vi "svx_Colormap Order lines.vi"(4 "pen":T1={"Width"=1, "Style"=enum."Solid"}, 5 "Order":dbl, 6 "color(black)":u32(colorbox), 7 "plot type":T2(ring), 8 "speed profile":cluster{"time [s]":dbl[], "speed [rpm]":dbl[]} {"speed [rpm]" format="%.2f"; "time [s]" format="%.2f"}, 9 "Range":T4, 10 "Plot area":T3, 11 "picture in":picture) -> (0 "End":cluster{"x":i16, "y":i16}, 2 "Begin":cluster{"x":i16, "y":i16}, 3 "picture out":picture)   [LabVIEW 2017, in "SVX Colormap.xctl"]
uses:
  <vilib>/addons/_XControls/Colormap/SVX Colormap.xctl
  <vilib>/Utility/miscctls.llb/LVBoundsTypeDef.ctl
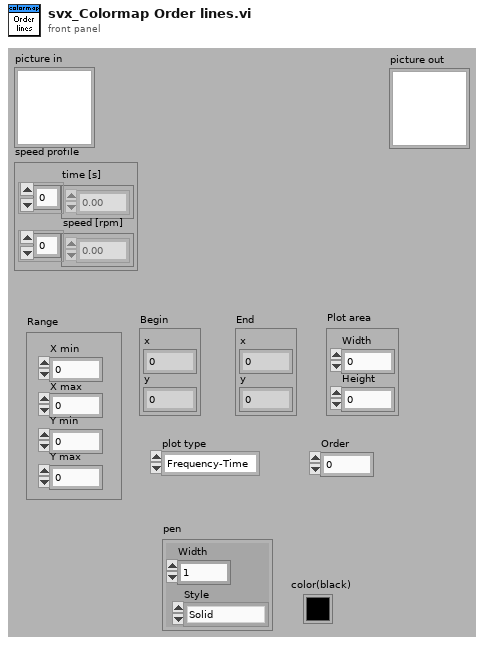
[diagram p1: front panel]
types:
  T1 = cluster{"Width":u16, "Style":enum32{"Solid", "Dash", "Dot", "DashDot", "DashDotDot"}}
  T2 = enum16{"Frequency-Time", "Time-Frequency", "Order-Time", "Time-Order", "Frequency-RPM", "RPM-Frequency", "Order-RPM", "RPM-Order"}
  T3 = typedef "LVBoundsTypeDef.ctl" = cluster{"Width":u32, "Height":u32}
  T4 = cluster{"X min":dbl, "X max":dbl, "Y min":dbl, "Y max":dbl}
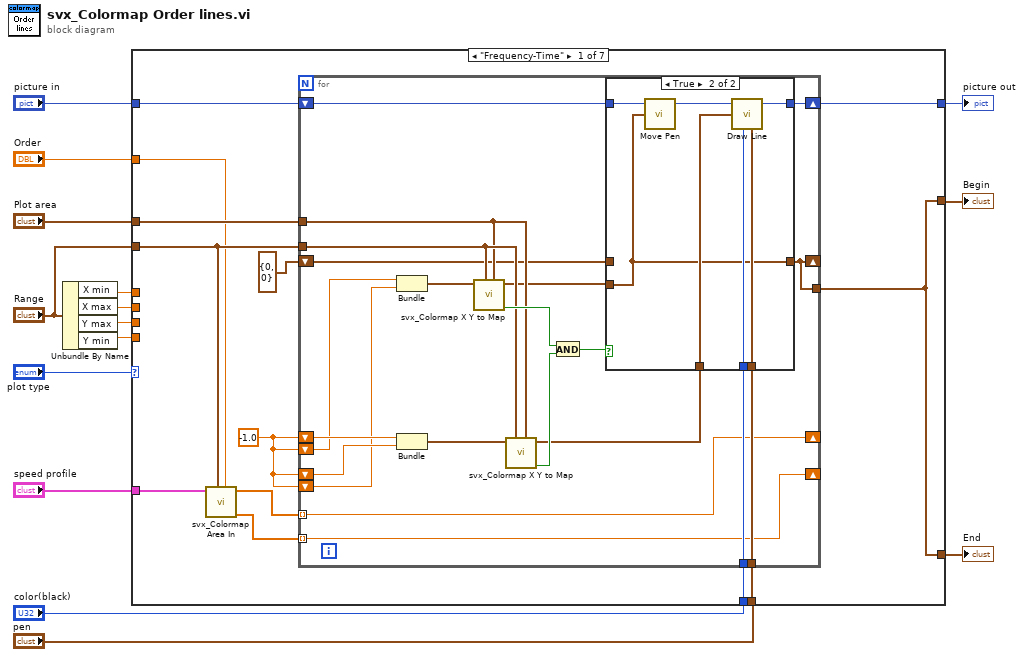
[diagram p0: block diagram]
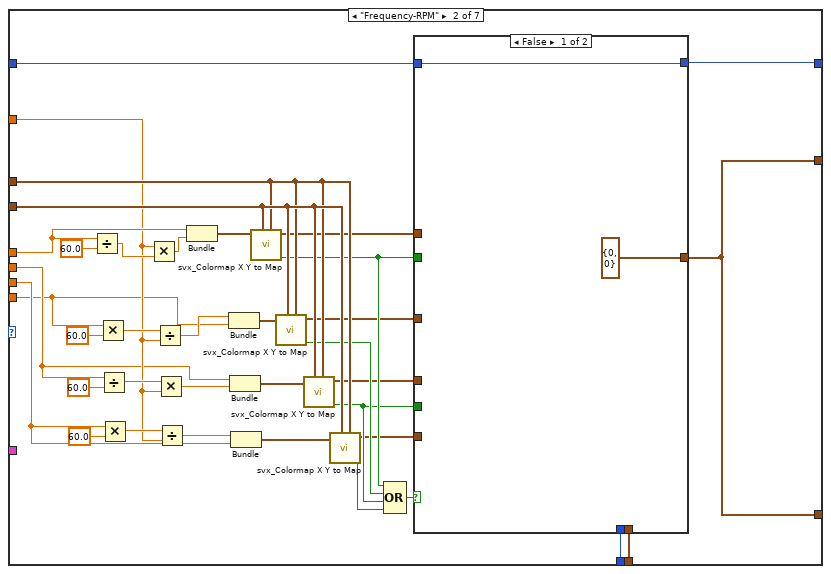
[diagram p3: hidden frame]
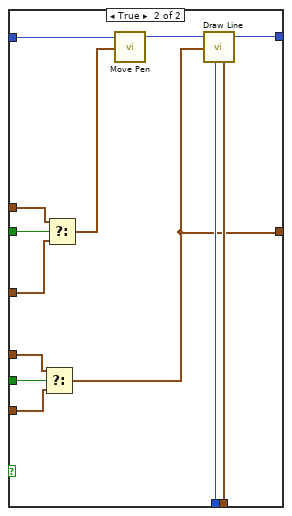
[diagram p4: hidden frame]
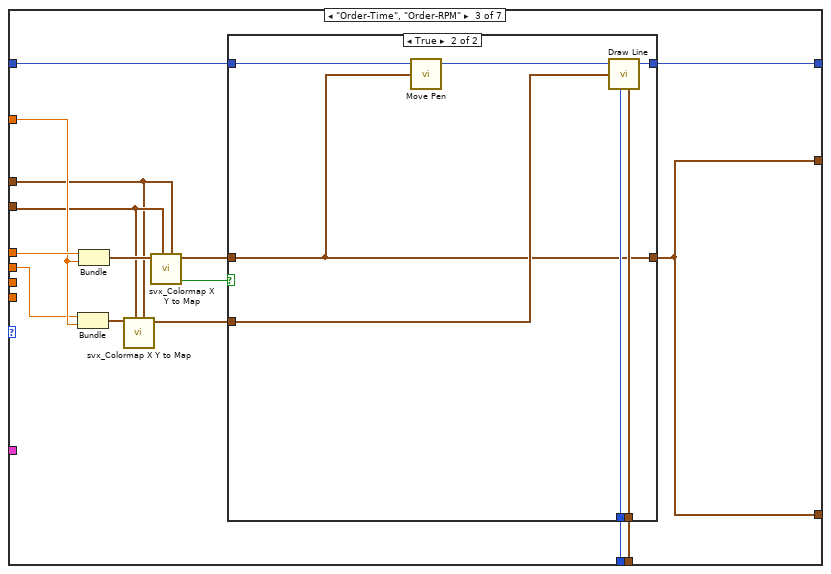
[diagram p5: hidden frame]
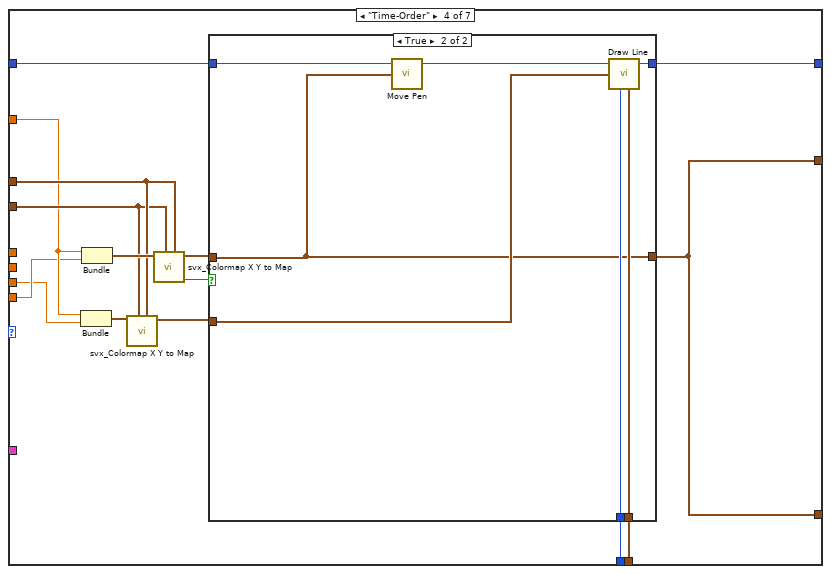
[diagram p7: hidden frame]
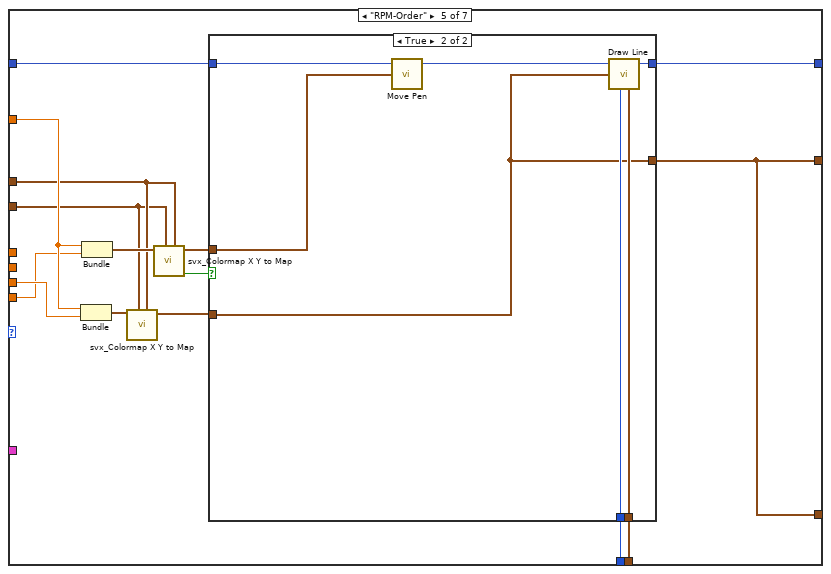
[diagram p9: hidden frame]
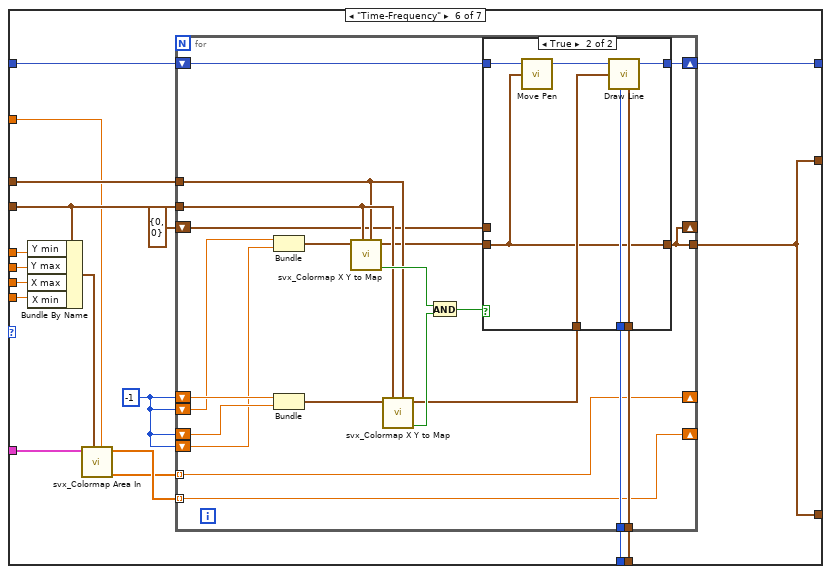
[diagram p11: hidden frame]
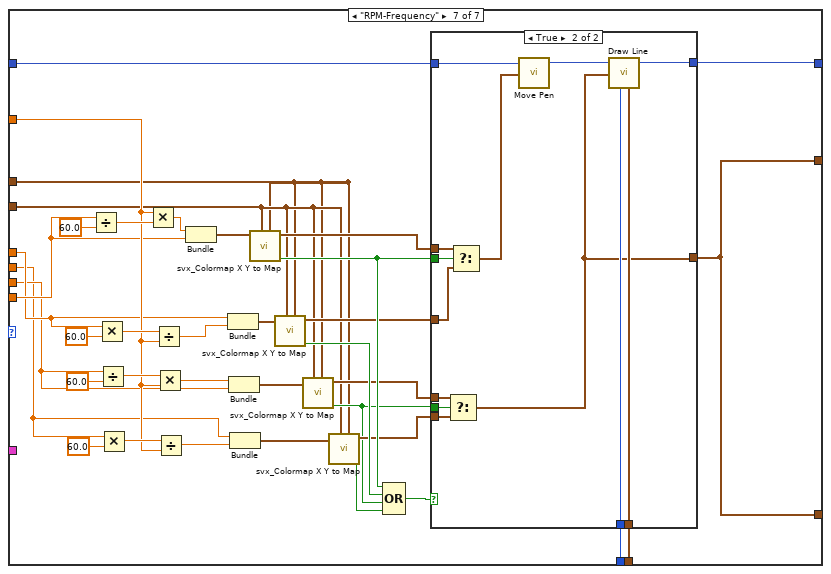
[diagram p13: hidden frame]
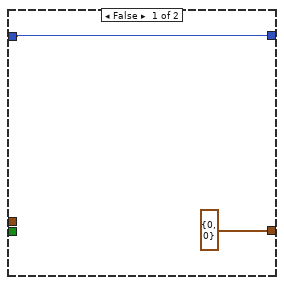
[diagram p14: hidden frame]
diagram:
  n1 = Unbundle By Name("Range") -> ("X min"=w8:dbl, "X max"=w13:dbl, "Y max"=w12:dbl, "Y min"=w11:dbl)
  n2 = case shown="\"Frequency-Time\"" "plot type" {
    tunnel: [w21 w66 w111 w135 w161 w188 w231] -> w15
    tunnel: [w21 w66 w111 w135 w161 w188 w231] -> w14
    tunnel: w8 -> [_ w95 w125 _ _ w193 w236]
    tunnel: w13 -> [_ w62 w116 _ _ w192 w233]
    tunnel: w12 -> [_ w81 _ w143 w160 w191 w234]
    tunnel: w11 -> [_ w59 _ w144 w159 w190 w237]
    tunnel: "Order" -> [w19 w64 w117 w145 w165 w185 w241]
    tunnel: "speed profile" -> [w17 _ _ _ _ w187 _]
    tunnel: "picture in" -> [w28 w75 w121 w141 w166 w200 w252]
    tunnel: [w27 w61 w122 w140 w162 w199 w251] -> w5
    tunnel: "color(black)" -> [w26 w74 w120 w137 w168 w196 w250]
    tunnel: "pen" -> [w25 w73 w119 w136 w167 w195 w249]
    tunnel: "Range" -> [w20 w80 w114 w146 w163 w194 w240]
    tunnel: "Plot area" -> [w24 w79 w113 w147 w164 w197 w239]
    frame "Frequency-Time" {
      w23 = -1.0 ("Numeric")
      n3 = call <vilib>:"svx_Colormap Area In.vi"("Order"=w19, "Range"=w20, "speed profile"=w17) -> ("Order"=w16:dbl[], "Time(s)"=w18:dbl[])  [unwired: 7 in]
      n4 = for {
        shift-right: [w46] -> w27
        shift-left: w28 -> [w45]
        tunnel: w16 -> [w31] mode=indexing
        tunnel: w18 -> [w32] mode=indexing
        tunnel: w26 -> [w44]
        tunnel: w25 -> [w43]
        tunnel: w20 -> [w42]
        tunnel: w24 -> [w41]
        shift-right: [w32] -> _
        shift-left: w23 -> [w40]
        shift-left: w23 -> [w39]
        shift-right: [w31] -> _
        shift-left: w23 -> [w38]
        shift-left: w23 -> [w37]
        shift-right: [w29] -> _
        shift-left: cluster{"x":i16, "y":i16} {"x"=0, "y"=0} ("Map") -> [w30]
        tunnel: [w29] -> w21
        n5 = Bundle("Numeric"=w39, "Numeric"=w37) -> (w36:cluster{"Numeric":dbl, "Numeric":dbl})  [unwired: 1 in]
        n6 = Bundle("Numeric"=w40, "Numeric"=w38) -> (w35:cluster{"Numeric":dbl, "Numeric":dbl})  [unwired: 1 in]
        n7 = call <vilib>:"svx_Colormap X Y to Map.vi"("Plot area"=w41, "Range"=w42, "cordinate"=w36) -> ("In?"=w48:bool, "Map"=w34:cluster{"x":i16, "y":i16})  [unwired: 7 in]
        n8 = call <vilib>:"svx_Colormap X Y to Map.vi"("Plot area"=w41, "Range"=w42, "cordinate"=w35) -> ("In?"=w49:bool, "Map"=w33:cluster{"x":i16, "y":i16})  [unwired: 7 in]
        n9 = And(x=w48, y=w49) -> (x .and. y?=w47:bool)
        n10 = case shown="True" w47 {
          tunnel: [w51 w56] -> w46
          tunnel: w45 -> [w51 w57]
          tunnel: w34 -> [_ w52]
          tunnel: w44 -> [_ w55]
          tunnel: w43 -> [_ w54]
          tunnel: w33 -> [_ w53]
          tunnel: w30 -> [w50 _]
          tunnel: [w50 w52] -> w29
          frame False {
          }
          frame True {
            n11 = call <vilib>:"Move Pen.vi"("new position"=w52, "picture"=w57) -> ("new picture"=w58:picture)  [unwired: 3 in]
            n12 = call <vilib>:"Draw Line.vi"("picture"=w58, "end point"=w53, "color(black)"=w55, "pen"=w54) -> ("new picture"=w56:picture)  [unwired: 5 in]
          }
        }
      }
    }
    frame "Frequency-RPM" {
      n13 = Divide(x=w95, y=60.0) -> (x/y=w92:dbl)
      n14 = Multiply(x=w59, y=60.0) -> (x*y=w65:dbl)
      n15 = Divide(x=w62, y=60.0) -> (x/y=w86:dbl)
      n16 = Multiply(x=w81, y=60.0) -> (x*y=w84:dbl)
      n17 = Multiply(x=w64, y=w92) -> (x*y=w91:dbl)
      n18 = Divide(x=w65, y=w64) -> (x/y=w60:dbl)
      n19 = Multiply(x=w86, y=w64) -> (x*y=w63:dbl)
      n20 = Divide(x=w84, y=w64) -> (x/y=w85:dbl)
      n21 = Bundle("X min"=w95, w91) -> (w93:cluster{"X min":dbl, dbl})  [unwired: 1 in]
      n22 = Bundle(w60, "Y min"=w59) -> (w89:cluster{dbl, "Y min":dbl})  [unwired: 1 in]
      n23 = Bundle("X max"=w62, w63) -> (w88:cluster{"X max":dbl, dbl})  [unwired: 1 in]
      n24 = Bundle(w85, "Y max"=w81) -> (w82:cluster{dbl, "Y max":dbl})  [unwired: 1 in]
      n25 = call <vilib>:"svx_Colormap X Y to Map.vi"("Plot area"=w79, "Range"=w80, "cordinate"=w93) -> ("In?"=w72:bool, "Map"=w71:cluster{"x":i16, "y":i16})  [unwired: 7 in]
      n26 = call <vilib>:"svx_Colormap X Y to Map.vi"("Plot area"=w79, "Range"=w80, "cordinate"=w89) -> ("In?"=w77:bool, "Map"=w70:cluster{"x":i16, "y":i16})  [unwired: 7 in]
      n27 = call <vilib>:"svx_Colormap X Y to Map.vi"("Plot area"=w79, "Range"=w80, "cordinate"=w88) -> ("In?"=w69:bool, "Map"=w68:cluster{"x":i16, "y":i16})  [unwired: 7 in]
      n28 = call <vilib>:"svx_Colormap X Y to Map.vi"("Plot area"=w79, "Range"=w80, "cordinate"=w82) -> ("In?"=w78:bool, "Map"=w67:cluster{"x":i16, "y":i16})  [unwired: 7 in]
      n29 = Compound Arithmetic op=OR(w72, w77, w69, w78) -> (w76:bool)
      n30 = case shown="False" w76 {
        tunnel: w75 -> [w97 w109]
        tunnel: w74 -> [_ w108]
        tunnel: w73 -> [_ w107]
        tunnel: [w97 w106] -> w61
        tunnel: w72 -> [_ w105]
        tunnel: w71 -> [_ w104]
        tunnel: w70 -> [_ w103]
        tunnel: w69 -> [_ w102]
        tunnel: w68 -> [_ w101]
        tunnel: w67 -> [_ w100]
        tunnel: [cluster{"x":i16, "y":i16} {"x"=0, "y"=0} ("Map") w98] -> w66
        frame False {
        }
        frame True {
          n31 = Select(t=w101, s=w102, f=w100) -> (s? t:f=w98:cluster{"x":i16, "y":i16})
          n32 = Select(t=w104, s=w105, f=w103) -> (s? t:f=w99:cluster{"x":i16, "y":i16})
          n33 = call <vilib>:"Move Pen.vi"("new position"=w99, "picture"=w109) -> ("new picture"=w110:picture)  [unwired: 3 in]
          n34 = call <vilib>:"Draw Line.vi"("picture"=w110, "end point"=w98, "color(black)"=w108, "pen"=w107) -> ("new picture"=w106:picture)  [unwired: 5 in]
        }
      }
    }
    frame "Order-Time", "Order-RPM" {
      n35 = Bundle("X max"=w116, "Order"=w117) -> (w115:cluster{"X max":dbl, "Order":dbl})  [unwired: 1 in]
      n36 = Bundle("X min"=w125, "Order"=w117) -> (w124:cluster{"X min":dbl, "Order":dbl})  [unwired: 1 in]
      n37 = call <vilib>:"svx_Colormap X Y to Map.vi"("Plot area"=w113, "Range"=w114, "cordinate"=w115) -> ("Map"=w112:cluster{"x":i16, "y":i16})  [unwired: 7 in, 1 out]
      n38 = call <vilib>:"svx_Colormap X Y to Map.vi"("Plot area"=w113, "Range"=w114, "cordinate"=w124) -> ("In?"=w123:bool, "Map"=w118:cluster{"x":i16, "y":i16})  [unwired: 7 in]
      n39 = case shown="True" w123 {
        tunnel: [w127 w133] -> w122
        tunnel: w121 -> [w127 w132]
        tunnel: w120 -> [_ w131]
        tunnel: w119 -> [_ w130]
        tunnel: w118 -> [_ w128]
        tunnel: w112 -> [w126 w129]
        tunnel: [w126 w128] -> w111
        frame False {
        }
        frame True {
          n40 = call <vilib>:"Move Pen.vi"("new position"=w128, "picture"=w132) -> ("new picture"=w134:picture)  [unwired: 3 in]
          n41 = call <vilib>:"Draw Line.vi"("picture"=w134, "end point"=w129, "color(black)"=w131, "pen"=w130) -> ("new picture"=w133:picture)  [unwired: 5 in]
        }
      }
    }
    frame "Time-Order" {
      n42 = Bundle("Order"=w145, "Y max"=w143) -> (w148:cluster{"Order":dbl, "Y max":dbl})  [unwired: 1 in]
      n43 = Bundle("Order"=w145, "Y min"=w144) -> (w149:cluster{"Order":dbl, "Y min":dbl})  [unwired: 1 in]
      n44 = call <vilib>:"svx_Colormap X Y to Map.vi"("Plot area"=w147, "Range"=w146, "cordinate"=w148) -> ("Map"=w138:cluster{"x":i16, "y":i16})  [unwired: 7 in, 1 out]
      n45 = call <vilib>:"svx_Colormap X Y to Map.vi"("Plot area"=w147, "Range"=w146, "cordinate"=w149) -> ("In?"=w142:bool, "Map"=w139:cluster{"x":i16, "y":i16})  [unwired: 7 in]
      n46 = case shown="True" w142 {
        tunnel: [w151 w157] -> w140
        tunnel: w141 -> [w151 w156]
        tunnel: w137 -> [_ w155]
        tunnel: w136 -> [_ w154]
        tunnel: w139 -> [_ w152]
        tunnel: w138 -> [w150 w153]
        tunnel: [w150 w152] -> w135
        frame False {
        }
        frame True {
          n47 = call <vilib>:"Move Pen.vi"("new position"=w152, "picture"=w156) -> ("new picture"=w158:picture)  [unwired: 3 in]
          n48 = call <vilib>:"Draw Line.vi"("picture"=w158, "end point"=w153, "color(black)"=w155, "pen"=w154) -> ("new picture"=w157:picture)  [unwired: 5 in]
        }
      }
    }
    frame "RPM-Order" {
      n49 = Bundle("Order"=w165, "Y max"=w160) -> (w172:cluster{"Order":dbl, "Y max":dbl})  [unwired: 1 in]
      n50 = Bundle("Order"=w165, "Y min"=w159) -> (w173:cluster{"Order":dbl, "Y min":dbl})  [unwired: 1 in]
      n51 = call <vilib>:"svx_Colormap X Y to Map.vi"("Plot area"=w164, "Range"=w163, "cordinate"=w172) -> ("Map"=w169:cluster{"x":i16, "y":i16})  [unwired: 7 in, 1 out]
      n52 = call <vilib>:"svx_Colormap X Y to Map.vi"("Plot area"=w164, "Range"=w163, "cordinate"=w173) -> ("In?"=w171:bool, "Map"=w170:cluster{"x":i16, "y":i16})  [unwired: 7 in]
      n53 = case shown="True" w171 {
        tunnel: [w175 w181] -> w162
        tunnel: w166 -> [w175 w180]
        tunnel: w168 -> [_ w179]
        tunnel: w167 -> [_ w178]
        tunnel: w170 -> [_ w177]
        tunnel: w169 -> [w174 w176]
        tunnel: [w174 w176] -> w161
        frame False {
        }
        frame True {
          n54 = call <vilib>:"Move Pen.vi"("new position"=w177, "picture"=w180) -> ("new picture"=w182:picture)  [unwired: 3 in]
          n55 = call <vilib>:"Draw Line.vi"("picture"=w182, "end point"=w176, "color(black)"=w179, "pen"=w178) -> ("new picture"=w181:picture)  [unwired: 5 in]
        }
      }
    }
    frame "Time-Frequency" {
      w198 = -1
      n56 = Bundle By Name(cluster=w194, "Y min"=w193, "Y max"=w192, "X max"=w191, "X min"=w190) -> (w186:T4)
      n57 = call <vilib>:"svx_Colormap Area In.vi"("Order"=w185, "Range"=w186, "speed profile"=w187) -> ("Order"=w183:dbl[], "Time(s)"=w184:dbl[])  [unwired: 7 in]
      n58 = for {
        shift-right: [w218] -> w199
        shift-left: w200 -> [w217]
        tunnel: w184 -> [w203] mode=indexing
        tunnel: w183 -> [w204] mode=indexing
        tunnel: w196 -> [w216]
        tunnel: w195 -> [w215]
        tunnel: w194 -> [w214]
        tunnel: w197 -> [w213]
        shift-right: [w204] -> _
        shift-left: w198 -> [w212]
        shift-left: w198 -> [w211]
        shift-right: [w203] -> _
        shift-left: w198 -> [w210]
        shift-left: w198 -> [w209]
        shift-right: [w201] -> _
        shift-left: cluster{"x":i16, "y":i16} {"x"=0, "y"=0} ("Map") -> [w202]
        tunnel: [w201] -> w188
        n59 = Bundle("Numeric"=w211, "Numeric"=w209) -> (w208:cluster{"Numeric":dbl, "Numeric":dbl})  [unwired: 1 in]
        n60 = Bundle("Numeric"=w212, "Numeric"=w210) -> (w207:cluster{"Numeric":dbl, "Numeric":dbl})  [unwired: 1 in]
        n61 = call <vilib>:"svx_Colormap X Y to Map.vi"("Plot area"=w213, "Range"=w214, "cordinate"=w208) -> ("In?"=w220:bool, "Map"=w206:cluster{"x":i16, "y":i16})  [unwired: 7 in]
        n62 = call <vilib>:"svx_Colormap X Y to Map.vi"("Plot area"=w213, "Range"=w214, "cordinate"=w207) -> ("In?"=w221:bool, "Map"=w205:cluster{"x":i16, "y":i16})  [unwired: 7 in]
        n63 = And(x=w220, y=w221) -> (x .and. y?=w219:bool)
        n64 = case shown="True" w219 {
          tunnel: [w223 w228] -> w218
          tunnel: w217 -> [w223 w229]
          tunnel: w206 -> [_ w224]
          tunnel: w216 -> [_ w227]
          tunnel: w215 -> [_ w226]
          tunnel: w205 -> [_ w225]
          tunnel: [w222 w224] -> w201
          tunnel: w202 -> [w222 _]
          frame False {
          }
          frame True {
            n65 = call <vilib>:"Move Pen.vi"("new position"=w224, "picture"=w229) -> ("new picture"=w230:picture)  [unwired: 3 in]
            n66 = call <vilib>:"Draw Line.vi"("picture"=w230, "end point"=w225, "color(black)"=w227, "pen"=w226) -> ("new picture"=w228:picture)  [unwired: 5 in]
          }
        }
      }
    }
    frame "RPM-Frequency" {
      n67 = Divide(x=w237, y=60.0) -> (x/y=w265:dbl)
      n68 = Multiply(x=w236, y=60.0) -> (x*y=w253:dbl)
      n69 = Divide(x=w234, y=60.0) -> (x/y=w259:dbl)
      n70 = Multiply(x=w233, y=60.0) -> (x*y=w258:dbl)
      n71 = Multiply(x=w241, y=w265) -> (x*y=w238:dbl)
      n72 = Divide(x=w253, y=w241) -> (x/y=w264:dbl)
      n73 = Multiply(x=w259, y=w241) -> (x*y=w235:dbl)
      n74 = Divide(x=w258, y=w241) -> (x/y=w232:dbl)
      n75 = Bundle(w238, "Y min"=w237) -> (w266:cluster{dbl, "Y min":dbl})  [unwired: 1 in]
      n76 = Bundle("X min"=w236, w264) -> (w262:cluster{"X min":dbl, dbl})  [unwired: 1 in]
      n77 = Bundle(w235, "Y max"=w234) -> (w261:cluster{dbl, "Y max":dbl})  [unwired: 1 in]
      n78 = Bundle("X max"=w233, w232) -> (w256:cluster{"X max":dbl, dbl})  [unwired: 1 in]
      n79 = call <vilib>:"svx_Colormap X Y to Map.vi"("Plot area"=w239, "Range"=w240, "cordinate"=w266) -> ("In?"=w247:bool, "Map"=w245:cluster{"x":i16, "y":i16})  [unwired: 7 in]
      n80 = call <vilib>:"svx_Colormap X Y to Map.vi"("Plot area"=w239, "Range"=w240, "cordinate"=w262) -> ("In?"=w254:bool, "Map"=w246:cluster{"x":i16, "y":i16})  [unwired: 7 in]
      n81 = call <vilib>:"svx_Colormap X Y to Map.vi"("Plot area"=w239, "Range"=w240, "cordinate"=w261) -> ("In?"=w242:bool, "Map"=w244:cluster{"x":i16, "y":i16})  [unwired: 7 in]
      n82 = call <vilib>:"svx_Colormap X Y to Map.vi"("Plot area"=w239, "Range"=w240, "cordinate"=w256) -> ("In?"=w255:bool, "Map"=w243:cluster{"x":i16, "y":i16})  [unwired: 7 in]
      n83 = Compound Arithmetic op=OR(w247, w254, w242, w255) -> (w248:bool)
      n84 = case shown="True" w248 {
        tunnel: w252 -> [w269 w281]
        tunnel: [w269 w280] -> w251
        tunnel: w250 -> [_ w279]
        tunnel: w249 -> [_ w278]
        tunnel: w247 -> [_ w277]
        tunnel: w246 -> [_ w276]
        tunnel: w245 -> [_ w275]
        tunnel: w244 -> [_ w274]
        tunnel: w243 -> [_ w273]
        tunnel: w242 -> [_ w272]
        tunnel: [cluster{"x":i16, "y":i16} {"x"=0, "y"=0} ("Map") w270] -> w231
        frame False {
        }
        frame True {
          n85 = Select(t=w274, s=w272, f=w273) -> (s? t:f=w270:cluster{"x":i16, "y":i16})
          n86 = Select(t=w275, s=w277, f=w276) -> (s? t:f=w271:cluster{"x":i16, "y":i16})
          n87 = call <vilib>:"Move Pen.vi"("new position"=w271, "picture"=w281) -> ("new picture"=w282:picture)  [unwired: 3 in]
          n88 = call <vilib>:"Draw Line.vi"("picture"=w282, "end point"=w270, "color(black)"=w279, "pen"=w278) -> ("new picture"=w280:picture)  [unwired: 5 in]
        }
      }
    }
  }
  "End" <- w14
  "Begin" <- w15
  "picture out" <- w5
